vi "FPGA_target_read_fifo.vi"(6 "data_in":T1, 7 "C0_in":T2, 8 "read_fifo":bool, 9 "C1_in":T2) -> (10 "fifo_empty":bool, 11 "C0_out":T2, 12 "data_out":T1, 13 "C1_out":T2)   [LabVIEW 2014]
doc: "Reads new data from the internal FIFO (or pipes the old data through)"
uses:
  FPGA_32BitPattern_data_type.ctl
  FPGA_cmd_data_type.ctl
  <vilib>/rvi/eio/common/nirviEmuReportErrorAndStop.vi
  <vilib>/rvi/errors/nirviReportUnexpectedCaseInternalError.vi
  <vilib>/rvi/errors/nirviReportUnexpectedCaseInternalError (U32).vi
  <vilib>/rvi/Emulation/niFpgaProcessEmulError.vi
  <vilib>/rvi/occurrence/nirviWaitOnOccurrenceBase.vi
  <vilib>/rvi/FIFO/Fifo_Resource/nirvififoEmulationReleaseLock.vi
  <vilib>/rvi/FIFO/Fifo_Resource/nirvififoEmulationObtainLock.vi
  <vilib>/rvi/FIFO/Fifo_Resource/nirvififoEmulationCreateLock.vi
  <vilib>/rvi/DataTransferAndStorage/Container/Common/niFpgaContainerGetUniqueNameForEmu.vi
  <vilib>/rvi/FIFO/Fifo_Resource/nirvififoEmulationSetSize.vi
  <vilib>/Utility/error.llb/Clear Errors.vi
  <vilib>/rvi/FIFO/Fifo_Resource/nirviFifoEmulationQueueMgr.vi
  <instcachedir>/0/nirviFifoEmulationQueueMgr_E5CAEC123FF24DC58D834DCA3CDAA9B5.lvgen/nirviFifoEmulationQueueMgr_E5CAEC123FF24DC58D834DCA3CDAA9B5_002.vi
  <vilib>/rvi/errors/niFpgaSetErrorForExecOnDevCompSimple.vi
  <vilib>/rvi/Emulation/niFpgaSctlEmulationGetInTimedLoop.vi
  <vilib>/rvi/Emulation/niFpgaEmulationIsFPGAContextNoSignature.vi
  <instcachedir>/0/nirviFifoEmulationQueueMgr_E5CAEC123FF24DC58D834DCA3CDAA9B5.lvgen/nirviFifoEmulationQueueMgr_E5CAEC123FF24DC58D834DCA3CDAA9B5_000.vi
  <vilib>/rvi/DataTransferAndStorage/Container/XNode/niFpgaContainer.xnode
  <vilib>/rvi/FIFO/Fifo_Resource/nirvififoEmulationRead.vi
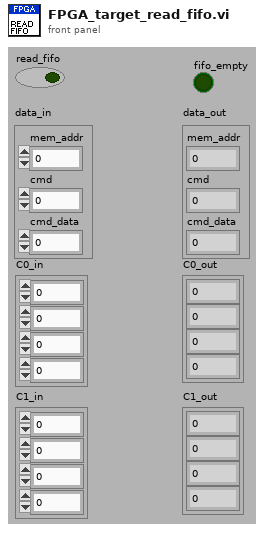
[diagram p1: front panel]
types:
  T1 = typedef "FPGA_cmd_data_type.ctl" = cluster{"mem_addr":u32, "cmd":u8, "cmd_data":u32}
  T2 = typedef "FPGA_32BitPattern_data_type.ctl" = cluster{"port0":u8, "port1":u8, "port2":u8, "port3":u8}
  T3 = cluster{"Element":u32, "Element":u8, "Element":u32}
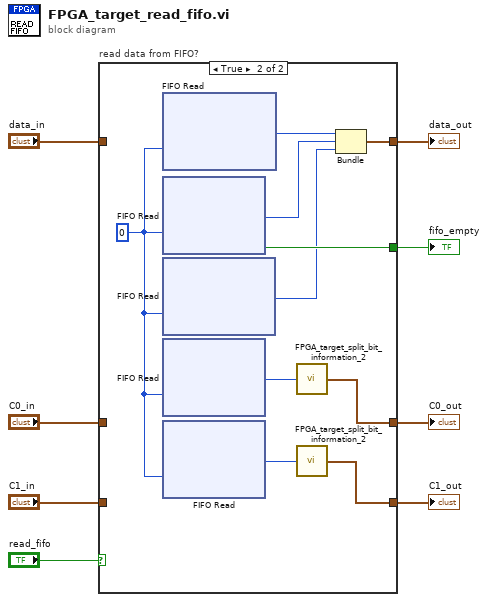
[diagram p0: block diagram]
diagram:
  n1 = case "read data from FIFO?" shown="True" "read_fifo" {
    selector: "read_fifo" -> [w10 _]
    tunnel: [w10 w22] -> w8
    tunnel: [w12 w21] -> w6
    tunnel: [w11 w18] -> w5
    tunnel: "C0_in" -> [w12 _]
    tunnel: "C1_in" -> [w11 _]
    tunnel: "data_in" -> [w9 _]
    tunnel: [w9 w17] -> w1
    frame False {
    }
    frame True {
      w13 = 0 ("Timeout")
      n2 = xnode ("FIFO Read")("Timeout"=w13) -> ("Element"=w14:u32)  [unwired: 1 in, 2 out]
      n3 = xnode ("FIFO Read")("Timeout"=w13) -> ("Element"=w16:u8, "Timed Out?"=w22:bool)  [unwired: 1 in, 1 out]
      n4 = xnode ("FIFO Read")("Timeout"=w13) -> ("Element"=w15:u32)  [unwired: 1 in, 2 out]
      n5 = xnode ("FIFO Read")("Timeout"=w13) -> ("Element"=w20:u32)  [unwired: 1 in, 2 out]
      n6 = xnode ("FIFO Read")("Timeout"=w13) -> ("Element"=w19:u32)  [unwired: 1 in, 2 out]
      n7 = call "FPGA_target_split_bit_information_2.vi"("data in"=w20) -> ("connector_data"=w21:T2)
      n8 = call "FPGA_target_split_bit_information_2.vi"("data in"=w19) -> ("connector_data"=w18:T2)
      n9 = Bundle("Element"=w14, "Element"=w16, "Element"=w15) -> (w17:T3)  [unwired: 1 in]
    }
  }
  "fifo_empty" <- w8
  "C0_out" <- w6
  "C1_out" <- w5
  "data_out" <- w1
